vi "RealTimeReadData.vi"(8 "error in":errorcluster, 11 "AllMotorReference(Same port)":T1[](array[typedef])) -> (0 "error out":errorcluster, 3 "ReadData":T4(array[cluster]))   [LabVIEW 2019, in "CubeMarsBLDClib.lvlib"]
uses:
  CubeMarsBLDClib.lvlib
  ReadMotorData.ctl
  Reference.ctl
  MotorType.ctl
panel:
  out "error count":i32
  out "Serial Settings:Number of Bytes at Serial Port":u32
  out "Read Data out":T3
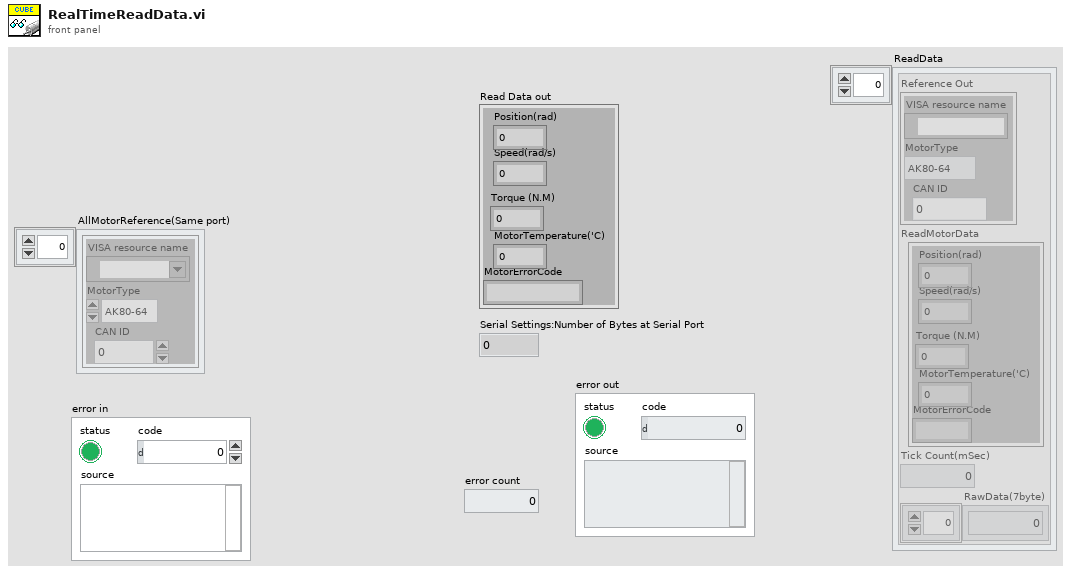
[diagram p1: front panel]
types:
  T1 = typedef "CubeMarsBLDClib.lvlib/Reference.ctl" = cluster{"VISA resource name":refnum<visa-resource-name>, "MotorType":T2, "CAN ID":u32}
  T2 = typedef "CubeMarsBLDClib.lvlib/MotorType.ctl" = enum16{"AK80-64", "AK80-9", "AK80-8", "AK80-6", "AK70-10", "AK60-6", "AK10-9"}
  T3 = typedef "CubeMarsBLDClib.lvlib/ReadMotorData.ctl" = cluster{"Position(rad)":dbl, "Speed(rad/s)":dbl, "Torque (N.M)":dbl, "MotorTemperature('C)":sgl, "MotorErrorCode":string}
  T4 = cluster{"Reference Out":T1, "ReadMotorData":T3, "Tick Count(mSec)":u32, "RawData(7byte)":u8[]}[]
  T5 = cluster{"Position(rad)":dbl, "Speed(rad/s)":dbl, "Kp":dbl}
  T6 = typedef "CubeMarsBLDClib.lvlib/MotorParameters.ctl" = cluster{"Position(rad)":dbl, "Speed(rad/s)":dbl, "Kp":dbl, "Kd":dbl, "Torque (N.M)":dbl}
  T7 = cluster{"Position(rad)":dbl, "Speed(rad/s)":dbl, "Torque (N.M)":dbl}
  T8 = cluster{"Reference Out":T1, "ReadMotorData":T3, "Tick Count(mSec)":u32, u8[]}
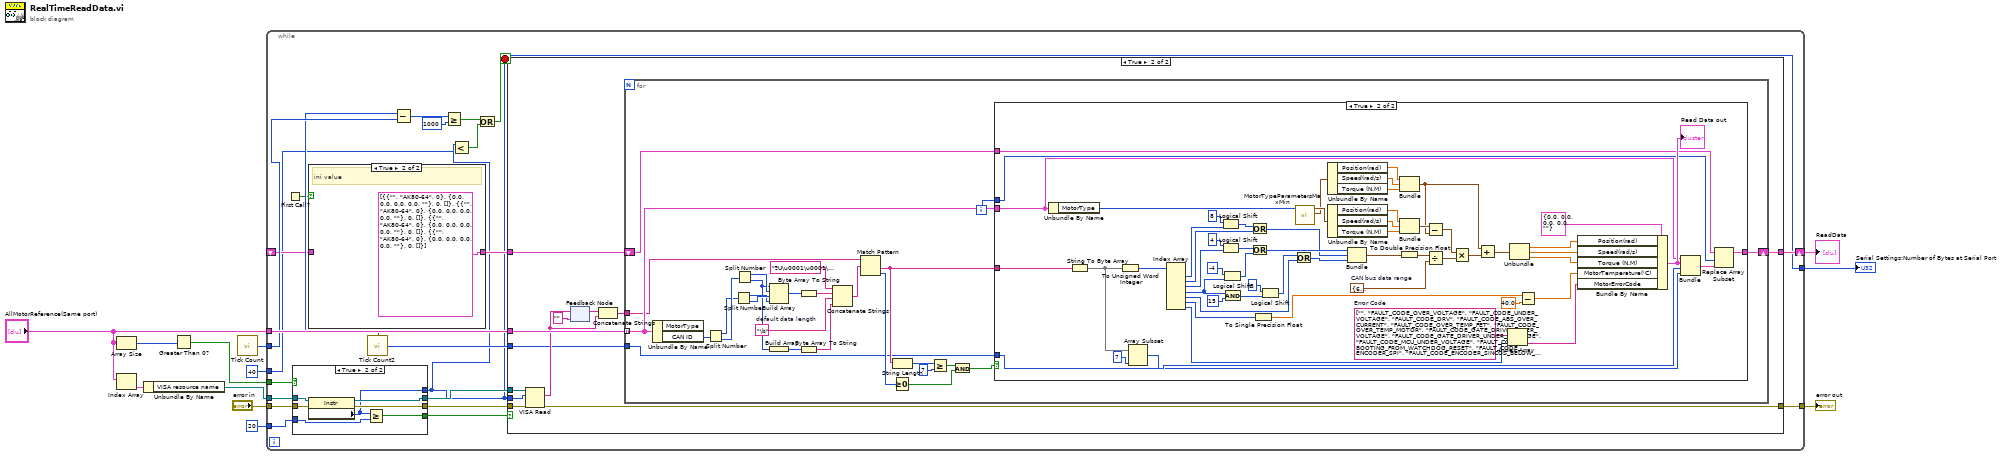
[diagram p0: block diagram]
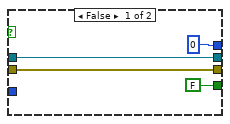
[diagram p3: hidden frame]
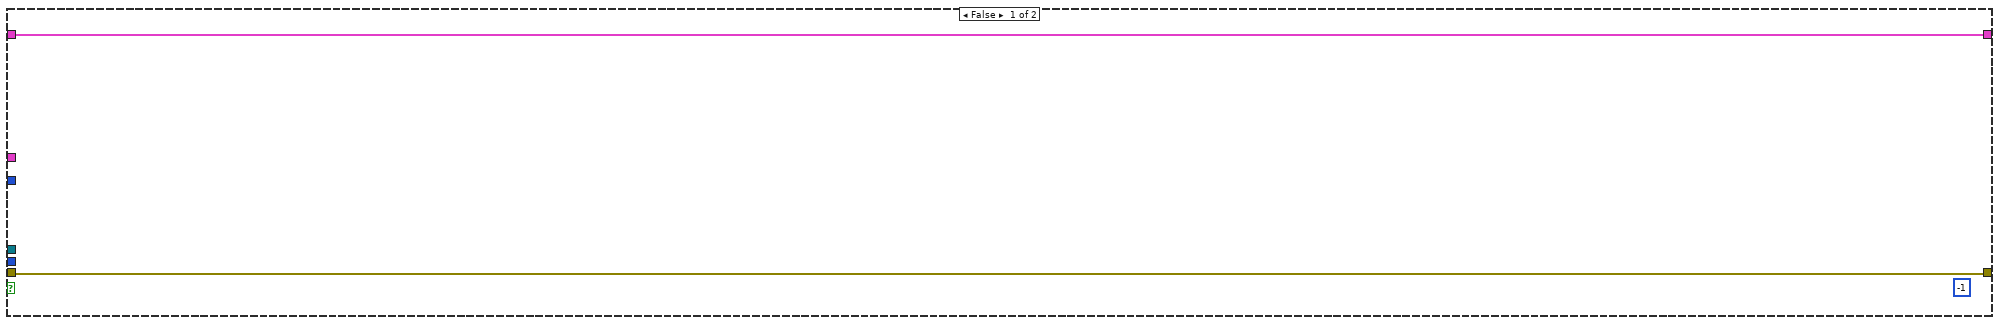
[diagram p4: hidden frame]
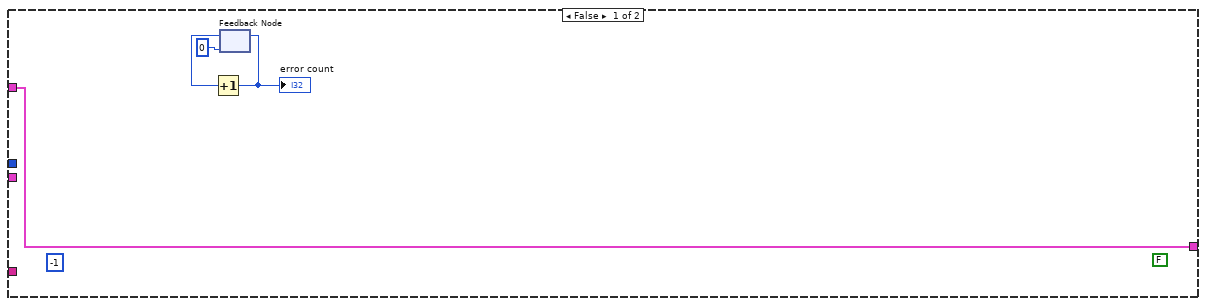
[diagram p5: hidden frame]
diagram:
  n1 = Array Size(array="AllMotorReference(Same port)") -> (size(s)=w3:i32)
  n2 = Index Array(array="AllMotorReference(Same port)") -> (element=w12:T1)  [unwired: 1 in]
  n3 = Unbundle By Name(w12) -> ("VISA resource name"=w11:refnum<visa-resource-name>)
  n4 = Greater Than 0?(x=w3) -> (x > 0?=w9:bool)
  n5 = call "Tick Count"() -> ("Tick Count(mSec)"=w4:u32)
  n6 = while {
    tunnel: w11 -> [w34]
    tunnel: "AllMotorReference(Same port)" -> [w33]
    tunnel: w9 -> [w30]
    tunnel: "error in" -> [w28]
    tunnel: w4 -> [w26]
    tunnel: u32 20 ("y") -> [w27]
    tunnel: u32 40 ("y") -> [w14]
    tunnel: [w15] -> w6
    shift-right: [w21] -> w5
    shift-left: _ -> [w19]
    tunnel: [w13] -> w1
    stop <- w22 stop-if-true
    n7 = First Call?() -> (First Call?: T/F=w18:bool)
    n8 = case shown="True" w30 {
      tunnel: w34 -> [w39 w47]
      tunnel: w28 -> [w40 w46]
      tunnel: [w40 w45] -> w32
      tunnel: [w39 w44] -> w31
      tunnel: w27 -> [_ w42]
      tunnel: [FALSE w43] -> w29
      tunnel: [u32 0 ("Bytes at Port") w41] -> w15
      frame False {
      }
      frame True {
        n9 = property class="Instr"(reference=w47, error in=w46) -> (reference out=w44:refnum<visa-resource-name>, error out=w45:errorcluster, "Serial Settings:Number of Bytes at Serial Port"=w41:u32)
        n10 = Greater Or Equal?(x=w41, y=w42) -> (x >= y?=w43:bool)
      }
    }
    n11 = case shown="True" w18 {
      tunnel: w19 -> [w35 _]
      tunnel: [w35 T4 [{"Reference Out"={"VISA resource name"="", "MotorType"=enum."AK80-64", "CAN ID"=0}, "ReadMotorData"={"Position(rad)"=0.0, "Speed(rad/s)"=0.0, "Torque (N.M)"=0.0, "MotorTemperature('C)"=0.0, "MotorErrorCode"=""}, "Tick Count(mSec)"=0, "RawData(7byte)"=[]}, {"Reference Out"={"VISA resource name"="", "MotorType"=enum."AK80-64", "CAN ID"=0}, "ReadMotorData"={"Position(rad)"=0.0, "Speed(rad/s)"=0.0, "Torque (N.M)"=0.0, "MotorTemperature('C)"=0.0, "MotorErrorCode"=""}, "Tick Count(mSec)"=0, "RawData(7byte)"=[]}, {"Reference Out"={"VISA resource name"="", "MotorType"=enum."AK80-64", "CAN ID"=0}, "ReadMotorData"={"Position(rad)"=0.0, "Speed(rad/s)"=0.0, "Torque (N.M)"=0.0, "MotorTemperature('C)"=0.0, "MotorErrorCode"=""}, "Tick Count(mSec)"=0, "RawData(7byte)"=[]}, {"Reference Out"={"VISA resource name"="", "MotorType"=enum."AK80-64", "CAN ID"=0}, "ReadMotorData"={"Position(rad)"=0.0, "Speed(rad/s)"=0.0, "Torque (N.M)"=0.0, "MotorTemperature('C)"=0.0, "MotorErrorCode"=""}, "Tick Count(mSec)"=0, "RawData(7byte)"=[]}]] -> w17
      frame False {
      }
      frame True {
        # "ini value"
      }
    }
    n12 = call "Tick Count2"() -> ("Tick Count(mSec)"=w20:u32)
    n13 = Subtract(x=w20, y=w26) -> (x-y=w16:u32)
    n14 = Greater Or Equal?(x=w16, y=u32 1000) -> (x >= y?=w23:bool)
    n15 = Less?(x=w15, y=w14) -> (x < y?=w24:bool)
    n16 = Compound Arithmetic op=OR(w23, w24) -> (w22:bool)
    n17 = case shown="True" w29 {
      tunnel: w33 -> [_ w61]
      tunnel: w32 -> [w49 w60]
      tunnel: w15 -> [_ w59]
      tunnel: w31 -> [_ w58]
      tunnel: [w49 w56] -> w13
      tunnel: w20 -> [_ w52]
      tunnel: [w48 w50] -> w21
      tunnel: w17 -> [w48 w51]
      frame False {
        (unwired) -1 ("CAN ID")
      }
      frame True {
        n18 = VISA Read(VISA resource name=w58, byte count=w59, error in (no error)=w60) -> (read buffer=w55:string, error out=w56:errorcluster)  [unwired: 2 out]
        n19 = feedback #1("" ("read buffer")) -> (w54:string)
        n20 = feedback-in #1(w55) -> ()
        n21 = Concatenate Strings(w54, w55) -> (w57:string)
        n22 = for {
          tunnel: w61 -> [w75] mode=indexing
          tunnel: w57 -> [w74]
          tunnel: w52 -> [w64]
          shift-right: [w62] -> w50
          shift-left: w51 -> [w63]
          i -> [w65]
          w77 = "\b"  # default data length
          n23 = Unbundle By Name(w75) -> ("CAN ID"=w76:u32)  [unwired: 1 out]
          n24 = Split Number(x=w76) -> (hi(x)=w86:u16, lo(x)=w87:u16)
          n25 = Split Number(x=w86) -> (hi(x)=w83:u8, lo(x)=w84:u8)
          n26 = Split Number(x=w87) -> (hi(x)=w85:u8, lo(x)=w79:u8)
          n27 = Build Array(w79, w85, w84, w83) -> (w82:u8[])
          n28 = Build Array(w79) -> (w80:u8[])
          n29 = Byte Array To String(unsigned byte array=w82) -> (string=w81:string)
          n30 = Byte Array To String(unsigned byte array=w80) -> (string=w78:string)
          n31 = Concatenate Strings("ªU\u0001\u0001\u0001" ("y"), w81, w77, w78) -> (w73:string)
          n32 = Match Pattern(string=w74, regular expression=w73) -> (after substring=w66:string, offset past match=w72:i32)  [unwired: 1 in, 2 out]
          n33 = Greater Or Equal To 0?(x=w72) -> (x >= 0?=w69:bool)
          n34 = String Length(string=w66) -> (length=w71:i32)
          n35 = Greater Or Equal?(x=w71, y=7) -> (x >= y?=w68:bool)
          n36 = And(x=w68, y=w69) -> (x .and. y?=w67:bool)
          n37 = case shown="True" w67 {
            tunnel: w75 -> [_ w98]
            tunnel: w66 -> [_ w103]
            tunnel: w65 -> [_ w94]
            tunnel: w64 -> [_ w99]
            tunnel: [w89 w96] -> w62
            tunnel: w63 -> [w89 w95]
            frame False {
              (unwired) -1 ("CAN ID")
              (unwired) FALSE
              n38 = feedback #2(0) -> (w91:i32)
              n39 = Increment(x=w91) -> (x+1=w92:i32)
              "error count" <- w92
              n40 = feedback-in #2(w92) -> ()
            }
            frame True {
              w122 = T5 {"Position(rad)"=65535.0, "Speed(rad/s)"=4095.0, "Kp"=4095.0}  # CAN bus data range
              w130 = string[] ["", "FAULT_CODE_OVER_VOLTAGE", "FAULT_CODE_UNDER_VOLTAGE", "FAULT_CODE_DRV", "FAULT_CODE_ABS_OVER_CURRENT", "FAULT_CODE_OVER_TEMP_FET", "FAULT_CODE_OVER_TEMP_MOTOR", "FAULT_CODE_GATE_DRIVER_OVER_VOLTAGE", "FAULT_CODE_GATE_DRIVER_UNDER_VOLTAGE", "FAULT_CODE_MCU_UNDER_VOLTAGE", "FAULT_CODE_BOOTING_FROM_WATCHDOG_RESET", "FAULT_CODE_ENCODER_SPI", "FAULT_CODE_ENCODER_SINCOS_BELOW_MIN_AMPLITUDE", "FAULT_CODE_ENCODER_SINCOS_ABOVE_MAX_AMPLITUDE", "FAULT_CODE_FLASH_CORRUPTION", "FAULT_CODE_HIGH_OFFSET_CURRENT_SENSOR_1", "FAULT_CODE_HIGH_OFFSET_CURRENT_SENSOR_2", "FAULT_CODE_HIGH_OFFSET_CURRENT_SENSOR_3", "FAULT_CODE_UNBALANCED_CURRENTS"]  # Error Code
              n41 = Unbundle By Name(w98) -> ("MotorType"=w135:T2)
              n42 = String To Byte Array(string=w103) -> (unsigned byte array=w102:u8[])
              n43 = To Unsigned Word Integer(number=w102) -> (unsigned 16bit integer=w146:u16[])
              n44 = Array Subset(array=w102, length=7) -> (w93:u8[])  [unwired: 1 in]
              n45 = Index Array(array=w146) -> (element #1=w144:u16, element #2=w145:u16, element #3=w151:u16, element #4=w141:u16, element #5=w136:u16, element #6=w134:u16, element #7=w129:u16)  [unwired: 7 in]
              n46 = Logical Shift(y=i16 8, x=w144) -> (x << y=w142:u16)
              n47 = Logical Shift(y=i16 4, x=w151) -> (x << y=w147:u16)
              n48 = Logical Shift(y=i16 -4, x=w141) -> (x << y=w148:u16)
              n49 = And(x=w141, y=u16 15) -> (x .and. y?=w139:u16)
              n50 = Or(x=w142, y=w145) -> (x .or. y?=w127:u16)
              n51 = Or(x=w147, y=w148) -> (x .or. y?=w126:u16)
              n52 = To Single Precision Float(number=w134) -> (single precision float=w133:sgl)
              n53 = Logical Shift(y=i16 8, x=w139) -> (x << y=w137:u16)
              n54 = Or(x=w137, y=w136) -> (x .or. y?=w125:u16)
              n55 = call "MotorTypeParametersMaxMin.vi"("MotorType"=w135) -> ("Min"=w113:T6, "Max"=w114:T6)  [unwired: 9 in]
              n56 = Unbundle By Name(w113) -> ("Position(rad)"=w117:dbl, "Speed(rad/s)"=w116:dbl, "Torque (N.M)"=w115:dbl)
              n57 = Unbundle By Name(w114) -> ("Position(rad)"=w120:dbl, "Speed(rad/s)"=w119:dbl, "Torque (N.M)"=w118:dbl)
              n58 = Bundle(w127, w126, w125) -> (w124:cluster{u16, u16, u16})  [unwired: 1 in]
              n59 = Bundle("Position(rad)"=w117, "Speed(rad/s)"=w116, "Torque (N.M)"=w115) -> (w109:T7)  [unwired: 1 in]
              n60 = Bundle("Position(rad)"=w120, "Speed(rad/s)"=w119, "Torque (N.M)"=w118) -> (w112:T7)  [unwired: 1 in]
              n61 = To Double Precision Float(number=w124) -> (double precision float=w123:cluster{dbl, dbl, dbl})
              n62 = Subtract(x=w112, y=w109) -> (x-y=w111:T7)
              n63 = Divide(x=w123, y=w122) -> (x/y=w121:cluster{dbl, dbl, dbl})
              n64 = Multiply(x=w111, y=w121) -> (x*y=w110:cluster{dbl, dbl, dbl})
              n65 = Add(x=w109, y=w110) -> (x+y=w108:cluster{dbl, dbl, dbl})
              n66 = Index Array(array=w130, index=w129) -> (element=w128:string)
              n67 = Unbundle(w108) -> (w107:dbl, w106:dbl, w105:dbl)
              n68 = Subtract(x=w133, y=sgl 40.0) -> (x-y=w131:sgl)
              n69 = Bundle By Name(cluster=T3 {"Position(rad)"=0.0, "Speed(rad/s)"=0.0, "Torque (N.M)"=0.0, "MotorTemperature('C)"=0.0, "MotorErrorCode"=""} ("ReadMotorData"), "Position(rad)"=w107, "Speed(rad/s)"=w106, "Torque (N.M)"=w105, "MotorTemperature('C)"=w131, "MotorErrorCode"=w128) -> (w100:T3)
              "Read Data out" <- w100
              n70 = Bundle("Reference Out"=w98, "ReadMotorData"=w100, "Tick Count(mSec)"=w99, w93) -> (w97:T8)  [unwired: 1 in]
              n71 = Replace Array Subset(array=w95, new element=w97, index=w94) -> (w96:T4)
            }
          }
        }
      }
    }
  }
  "Serial Settings:Number of Bytes at Serial Port" <- w6
  "error out" <- w1
  "ReadData" <- w5
